vi "Setup GAS TestRunner.vi"(4 "Exclude Bookmarks":string[](array[string]), 5 "Verbose":bool, 6 "Include Bookmarks":string[](array[string]), 7 "CLI":refnum<class "CLI.lvclass">, 8 "error in (no error)":errorcluster, 9 "Report Path":path, 10 "Paths":path[](array[path]), 11 "DMC Test Runner.Folder":refnum<class "DMC Test Runner.lvclass">) -> (0 "error out":errorcluster, 3 "DMC Test Runner.Folder out":refnum<class "DMC Test Runner.lvclass">)   [LabVIEW 2023, in "DMC Test Runner.lvclass"]
uses:
  DMC Test Runner.lvclass
  C:/Program Files/National Instruments/LabVIEW 2023/vi.lib/addons/_JKI Toolkits/Caraya/classes/Test Runner/Test Runner.lvclass
  <vilib>/Wiresmith Technology/G CLI/CLI Class/CLI.lvclass
  <vilib>/addons/_JKI Toolkits/Caraya/classes/Test Runner/Test Runner.lvclass/Test Runner.ctl
  DMC Test Runner.lvclass/DMC Test Runner.ctl
  <vilib>/addons/_JKI Toolkits/Caraya/classes/Test Runner/Test Runner.lvclass
  <vilib>/addons/_JKI Toolkits/Caraya/Caraya.lvlib
  C:/projects/DMC/GitHub/DMC CLI Caraya/Source/DMC Test Runner/DMC Test Runner.lvclass
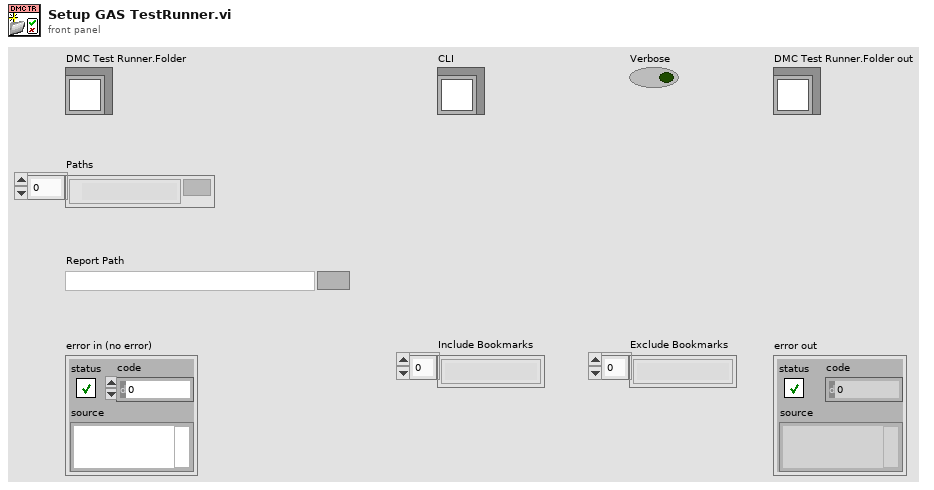
[diagram p1: front panel]
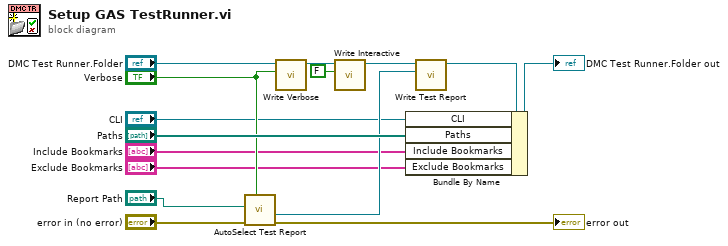
[diagram p0: block diagram]
diagram:
  n1 = call <vilib>:"AutoSelect Test Report.vi"("Verbose"="Verbose", "error in (no error)"="error in (no error)", "Report Path"="Report Path") -> ("error out"=→"error out":errorcluster, "Test Report out"=w9:refnum<class "Test Report.lvclass">)  [unwired: 7 in]
  n2 = call <vilib>:"Write Verbose.vi"("Verbose"="Verbose", "Test Runner in"="DMC Test Runner.Folder") -> ("Test Runner out"=w11:refnum<class "DMC Test Runner.lvclass">)  [unwired: 9 in]
  n3 = call <vilib>:"Write Interactive.vi"("Interactive"=FALSE, "Test Runner in"=w11) -> ("Test Runner out"=w10:refnum<class "DMC Test Runner.lvclass">)  [unwired: 9 in]
  n4 = call <vilib>:"Write Test Report.vi"("Test Report"=w9, "Test Runner in"=w10) -> ("Test Runner out"=w15:refnum<class "DMC Test Runner.lvclass">)  [unwired: 9 in]
  n5 = Bundle By Name(cluster=w15, "CLI"="CLI", "Paths"="Paths", "Include Bookmarks"="Include Bookmarks", "Exclude Bookmarks"="Exclude Bookmarks") -> (→"DMC Test Runner.Folder out":refnum<class "DMC Test Runner.lvclass">)
